vi "DCA Convert T-F to HTML.vi"(10 "(T/F)":bool) -> (2 "HTML (true/false)":string)   [LabVIEW 2011]
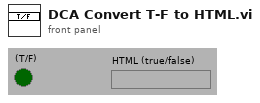
[diagram p1: front panel]
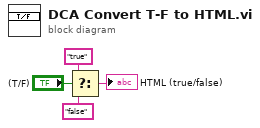
[diagram p0: block diagram]
diagram:
  n1 = Select(t="true" ("format string"), s="(T/F)", f="false" ("format string")) -> (s? t:f=→"HTML (true/false)":string)
